vi "NIFPGA-MCS.reset.vi"(0 "i ref in":refnum<vi>, 5 "error in (no error)":errorcluster) -> (14 "i ref out":refnum<vi>, 19 "error out":errorcluster)   [LabVIEW 2014, in "NIFPGA-MCS.lvlib"]
doc: "Resets the MCS to its default value. Calling this function might cause an \"empty run\" of the MCS, in case the MCS has been waiting for a start trigger."
uses:
  NIFPGA-MCS.lvlib
  CSCore/CSApplicationBaseClasses/MCSBase/MCSBase.statusType.ctl
  CSlibraries/UtilityLib/UtilityLib.valueStatus.ctl
  CSCore/CSApplicationBaseClasses/DeviceBase/DeviceBase.lvlib
  CSinstr.lib/NI-FPGA-MCS/host/instrumentDriver/NI-FPGA-MCS_Driver.lvlib
  CSCore/CSApplicationBaseClasses/MCSBase/MCSBase.lvlib
  CSlibraries/UtilityLib/UtilityLib.lvlib
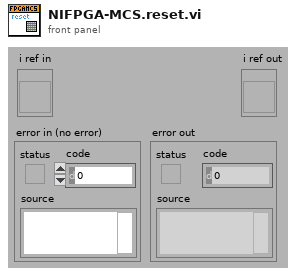
[diagram p1: front panel]
types:
  T1 = typedef "UtilityLib.lvlib/UtilityLib.valueStatus.ctl" = enum16{"no info available", "stand by/off", "on", "warning", "alarm/malfunction", "not implemented", "user action required", "important information", "system default", "control default", "indicator default", "button default"}
  T2 = typedef "MCSBase.lvlib/MCSBase.statusType.ctl" = i32
  T3 = typedef "NIFPGA-MCS.lvlib/NIFPGA-MCS.i attribute.ctl" = cluster{"fpgaViRef":T4}
  T4 = typedef "NI-FPGA-MCS_Driver.lvlib/fpga_vi_ref.ctl" = refnum<k20>
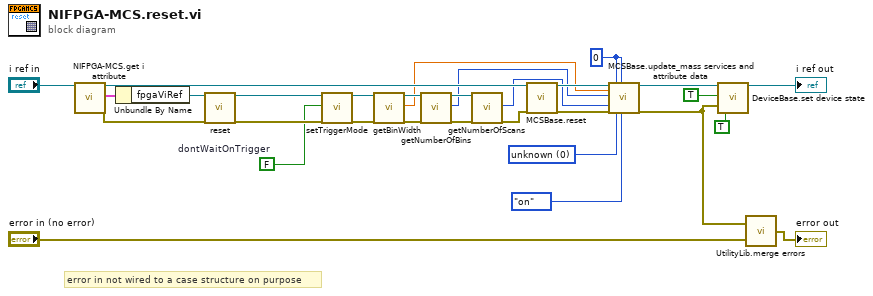
[diagram p0: block diagram]
diagram:
  w4 = FALSE  # dontWaitOnTrigger
  w19 = T2 0 items=["unknown"=0, "configured"=1, "error"=32] ("status")
  w20 = 0 ("totalCounts")
  # "error in not wired to a case structure on purpose"
  n1 = call "NIFPGA-MCS.get i attribute.vi"("i ref in"="i ref in") -> ("i ref out"=w24:refnum<vi>, "i attribute"=w27:T3, "error out"=w28:errorcluster)  [unwired: 16 in]
  n2 = Unbundle By Name(w27) -> ("fpgaViRef"=w25:T4)
  n3 = call "reset.vi"("fpga_vi_ref"=w25, "error in (no error)"=w28) -> ("fpga_vi_ref out"=w8:T4, "error out"=w5:errorcluster)  [unwired: 15 in, 1 out]
  n4 = call "setTriggerMode.vi"("fpga_vi_ref"=w8, "dontWaitOnTrigger (FALSE)"=w4, "error in (no error)"=w5) -> ("fpga_vi_ref out"=w7:T4, "error out"=w6:errorcluster)  [unwired: 15 in]
  n5 = call "getBinWidth.vi"("fpga_vi_ref"=w7, "error in (no error)"=w6) -> ("fpga_vi_ref out"=w17:T4, "binWidth [us]"=w12:dbl, "error out"=w15:errorcluster)  [unwired: 15 in]
  n6 = call "getNumberOfBins.vi"("fpga_vi_ref"=w17, "error in (no error)"=w15) -> ("fpga_vi_ref out"=w16:T4, "nOfBins"=w11:u16, "error out"=w14:errorcluster)  [unwired: 15 in]
  n7 = call "getNumberOfScans.vi"("fpga_vi_ref"=w16, "error in (no error)"=w14) -> ("nOfScans"=w10:u32, "error out"=w13:errorcluster)  [unwired: 15 in, 1 out]
  n8 = call "MCSBase.reset.vi"("i ref in"=w24, "error in (no error)"=w13) -> ("i ref out"=w22:refnum<vi>, "error out"=w23:errorcluster)  [unwired: 16 in]
  n9 = call "MCSBase.update_mass services and attribute data.vi"("i ref in"=w22, "binWidth [us]"=w12, "nOfBins"=w11, "nOfRecords"=w10, "error in (no error)"=w23, "counts"=w20, "status"=w19, "totalCounts"=w20, "valueStatus"=UtilityLib.valueStatus."on") -> ("i ref out"=w21:refnum<vi>, "error out"=w2:errorcluster)  [unwired: 8 in, 1 out]
  n10 = call "DeviceBase.set device state.vi"("i ref in"=w21, "implicit"=TRUE, "device error"=w2, "mayResetError (FALSE)"=TRUE) -> ("i ref out"=→"i ref out":refnum<vi>)  [unwired: 13 in, 2 out]
  n11 = call "UtilityLib.merge errors.vi"("error2 (no error)"="error in (no error)", "error1 (no error)"=w2) -> ("error out"=→"error out":errorcluster)
